vi "How many bytes to look for.vi"(10 "x":i64, 11 "Numeric in":i32) -> (3 "Numeric out":i64)   [LabVIEW 2012]
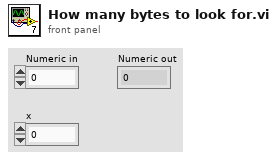
[diagram p1: front panel]
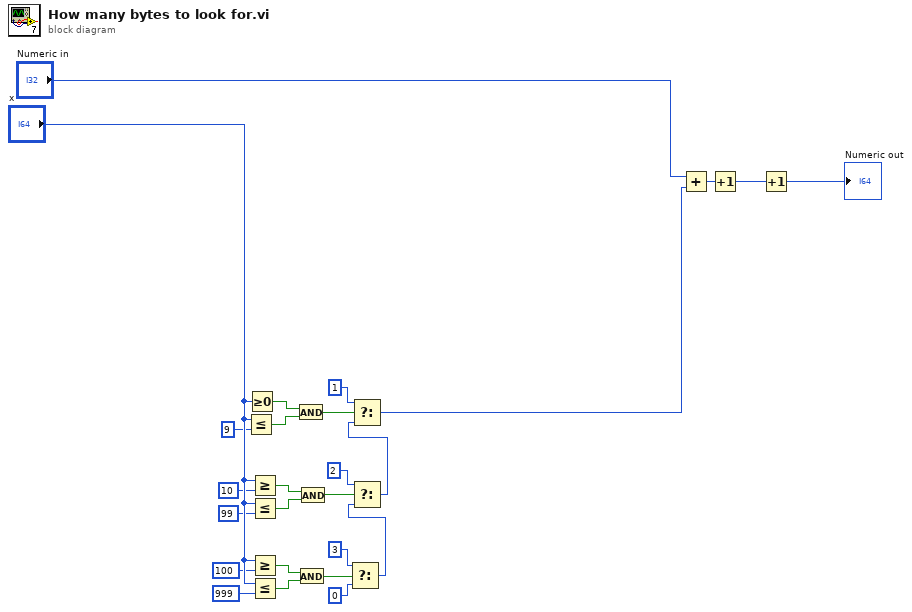
[diagram p0: block diagram]
diagram:
  n1 = Less Or Equal?(x="x", y=i64 9) -> (x <= y?=w12:bool)
  n2 = Greater Or Equal To 0?(x="x") -> (x >= 0?=w7:bool)
  n3 = Greater Or Equal?(x="x", y=i64 10) -> (x >= y?=w11:bool)
  n4 = Less Or Equal?(x="x", y=i64 99) -> (x <= y?=w10:bool)
  n5 = Greater Or Equal?(x="x", y=i64 100) -> (x >= y?=w9:bool)
  n6 = Less Or Equal?(x="x", y=i64 999) -> (x <= y?=w8:bool)
  n7 = And(x=w7, y=w12) -> (x .and. y?=w13:bool)
  n8 = And(x=w9, y=w8) -> (x .and. y?=w15:bool)
  n9 = And(x=w11, y=w10) -> (x .and. y?=w14:bool)
  n10 = Select(t=i64 3 ("y"), s=w15, f=i64 0) -> (s? t:f=w20:i64)
  n11 = Select(t=i64 2 ("y"), s=w14, f=w20) -> (s? t:f=w19:i64)
  n12 = Select(t=i64 1 ("y"), s=w13, f=w19) -> (s? t:f=w22:i64)
  n13 = Add(x="Numeric in", y=w22) -> (x+y=w23:i64)
  n14 = Increment(x=w23) -> (x+1=w26:i64)
  n15 = Increment(x=w26) -> (x+1=→"Numeric out":i64)
